vi "Main Project That Uses SubVI.vi"() -> ()   [LabVIEW 2024]
panel:
  out "F":dbl
  in  "r":dbl
  in  "q2":dbl
  in  "q1":dbl
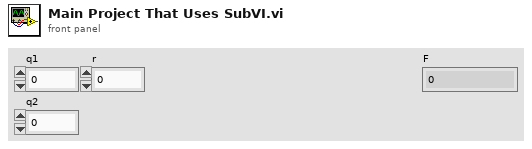
[diagram p1: front panel]
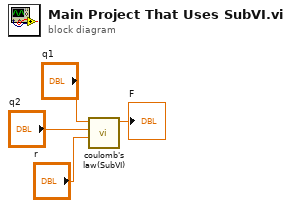
[diagram p0: block diagram]
diagram:
  n1 = call "coulomb's law(SubVI).vi"("r"="r", "q2"="q2", "q1"="q1") -> ("F"=→"F":dbl)  [unwired: 8 in]
